vi "GamePad Drive.vi"   [LabVIEW 2013]
uses:
  Team Code/Robot Global Data.vi
types:
  T1 = typedef "Gamepad.ctl" = cluster{"Buttons":T2, "Axes":cluster{"axis 1 (x)":dbl, "axis 2 (y)":dbl, "axis 3 (throttle)":dbl, "axis 4":dbl, "axis 5":dbl, "axis 6":dbl}}
  T2 = typedef "WPI_JoystickButtonState.ctl" = cluster{"Button 1":bool, "Button 2":bool, "Button 3":bool, "Button 4":bool, "Button 5":bool, "Button 6":bool, "Button 7":bool, "Button 8":bool, "Button 9":bool, "Button 10":bool, "Button 11":bool, "Button 12":bool}
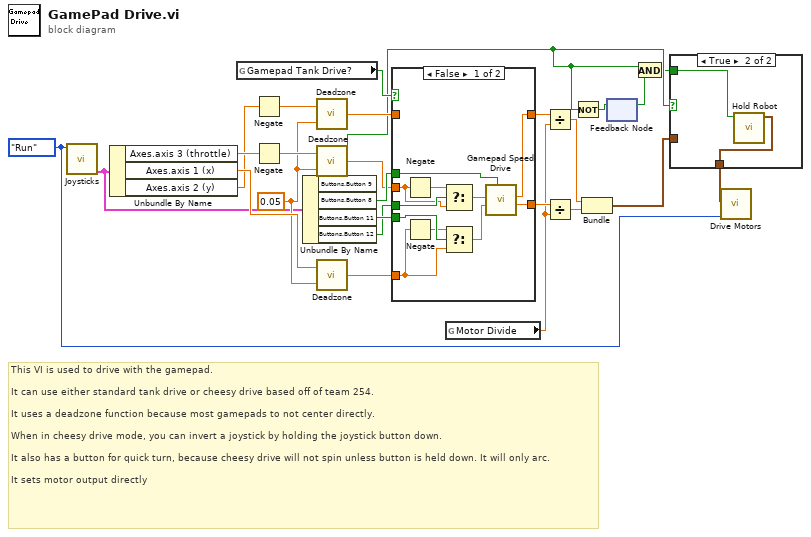
[diagram p0: block diagram]
diagram:
  w17 = 0.05 ("Deadzone")
  w26 = enum16{"Init", "Run", "End"}."Run" ("Mode")
  # "This VI is used to drive with the gamepad. \n\nIt can use either standard tank drive or cheesy drive based off of team 254.\n\nIt uses a deadzone function because most gamepads to not center directly.\n\nWhen in cheesy drive mode, you can invert a joystick by holding the joystick button down.\n\nIt also has a button for quick turn, because cheesy drive will not spin unless button is held down. It will only arc.\n\nIt sets motor output directly"
  n1 = call "Joysticks.vi"("Mode"=w26) -> ("GamePad"=w13:T1)  [unwired: 8 out]
  n2 = Unbundle By Name(w13) -> ("Axes.axis 3 (throttle)"=w24:dbl, "Axes.axis 1 (x)"=w25:dbl, "Axes.axis 2 (y)"=w15:dbl)
  n3 = global read "Robot Global Data.vi" "Gamepad Tank Drive?"() -> (w10:bool)
  n4 = Negate(x=w15) -> (-x=w14:dbl)
  n5 = Negate(x=w24) -> (-x=w23:dbl)
  n6 = Unbundle By Name(w13) -> ("Buttons.Button 9"=w4:bool, "Buttons.Button 8"=w22:bool, "Buttons.Button 11"=w9:bool, "Buttons.Button 12"=w8:bool)
  n7 = call "Deadzone.vi"("Deadzone"=w17, "Input"=w14) -> ("Output"=w16:dbl)
  n8 = call "Deadzone.vi"("Deadzone"=w17, "Input"=w23) -> ("Output"=w21:dbl)
  n9 = call "Deadzone.vi"("Deadzone"=w17, "Input"=w25) -> ("Output"=w20:dbl)
  n10 = case shown="False" w10 {
    tunnel: w22 -> [w31 _]
    tunnel: w21 -> [w28 w38]
    tunnel: w20 -> [w33 _]
    tunnel: [w37 w39] -> w19
    tunnel: [w36 w38] -> w18
    tunnel: w16 -> [_ w39]
    tunnel: w9 -> [w35 _]
    tunnel: w8 -> [w30 _]
    frame False {
      n11 = Negate(x=w28) -> (-x=w29:dbl)
      n12 = Negate(x=w33) -> (-x=w34:dbl)
      n13 = Select(t=w29, s=w30, f=w28) -> (s? t:f=w27:dbl)
      n14 = Select(t=w34, s=w35, f=w33) -> (s? t:f=w32:dbl)
      n15 = call "Gamepad Speed Drive.vi"("Quick Turn"=w31, "Turn"=w32, "Speed"=w27) -> ("Right Output"=w36:dbl, "Left Output"=w37:dbl)  [unwired: 7 out]
    }
    frame True {
    }
  }
  n16 = global read "Robot Global Data.vi" "Motor Divide"() -> (w7:dbl)
  n17 = Divide(x=w19, y=w7) -> (x/y=w12:dbl)
  n18 = Divide(x=w18, y=w7) -> (x/y=w11:dbl)
  n19 = Not(x=w4) -> (.not. x?=w6:bool)
  n20 = Bundle(w12, w11) -> (w1:cluster{dbl, dbl})  [unwired: 1 out]
  n21 = feedback #1() -> (w5:bool)  [unwired: 1 in]
  n22 = feedback-in #1(w6) -> ()
  n23 = And(x=w4, y=w5) -> (x .and. y?=w3:bool)
  n24 = case shown="True" w4 {
    tunnel: w3 -> [_ w42]
    tunnel: [w40 w41] -> w2
    tunnel: w1 -> [w40 _]
    frame False {
    }
    frame True {
      n25 = call "Hold Robot.vi"("Reset Encoders?"=w42) -> ("Speed Output"=w41:cluster{"output":dbl, "output":dbl})  [unwired: 10 in]
    }
  }
  n26 = call "Drive Motors.vi"("Mode"=w26, "Inputs"=w2) -> ()  [unwired: 2 in, 8 out]
